vi "read_db_for_plot.vi"(8 "error in (no error)":errorcluster, 11 "Constraints 2":T1={"Upper Timestamp Range"=timestamp(0 s since 1904-01-01), "Lower Timestamp Range"=timestamp(0 s since 1904-01-01), "Experiment Group:"="", "Experiment Name:"=[], "Upper Velocity Limit (km/s)"=0.0, "Lower Velocity Limit (km/s)"=0.0, "Upper Mass Limit (kg)"=0.0, "Lower Mass Limit (kg)"=0.0, "Estimate Source "=-2, "name array"=[]} {"Estimate Source" items=["Any Source."=-2, "No Shot"=-1, "Basic Labview Estimate"=0, "IDL Estimate From Andrew"=1, "IDL Estimate From Tobin"=2, "Old Metadata"=3]}) -> (0 "error out":errorcluster, 1 "Total Number of events":i64, 2 "Dust Event ID Array":i64[](array[numeric]), 3 "Dust Array":T3[](array[typedef]) {"File Location" items=["Currently Writing"=-3, "Labview Files"=-2, "Mars Data Processing Factility"=-1, "Local Cache "=0, "Old Storage"=1, "Storage"=2]; "Estimate Source" items=["Any Source."=-2, "No Shot"=-1, "Basic Labview Estimate"=0, "IDL Estimate From Andrew"=1, "IDL Estimate From Tobin"=2, "Old Metadata"=3]}, 4 "Dust Info":cluster{"Density":dbl, "Name":string}[](array[cluster]))   [LabVIEW 2012]
uses:
  Public API/Query_Dust_Event.ctl
  Estimate_source.ctl
  File_location.ctl
  Constraints.ctl
  <vilib>/addons/database/Auxilliary.llb/DB Tools Cursor Type.ctl
  <vilib>/addons/database/Connection.llb/Conn Execute.vi
  <vilib>/addons/database/Recordset.llb/Rec Fetch Recordset Data (R).vi
  <vilib>/addons/database/Recordset.llb/Rec Destroy - Connection.vi
  <vilib>/addons/database/_DB Variant To Data/Database Variant To Data.xnode
  <vilib>/addons/database/NI_Database_API.lvlib
panel:
  out "resulting string":string
  out "SQL Query Sintax":string
  # "Dust Event"
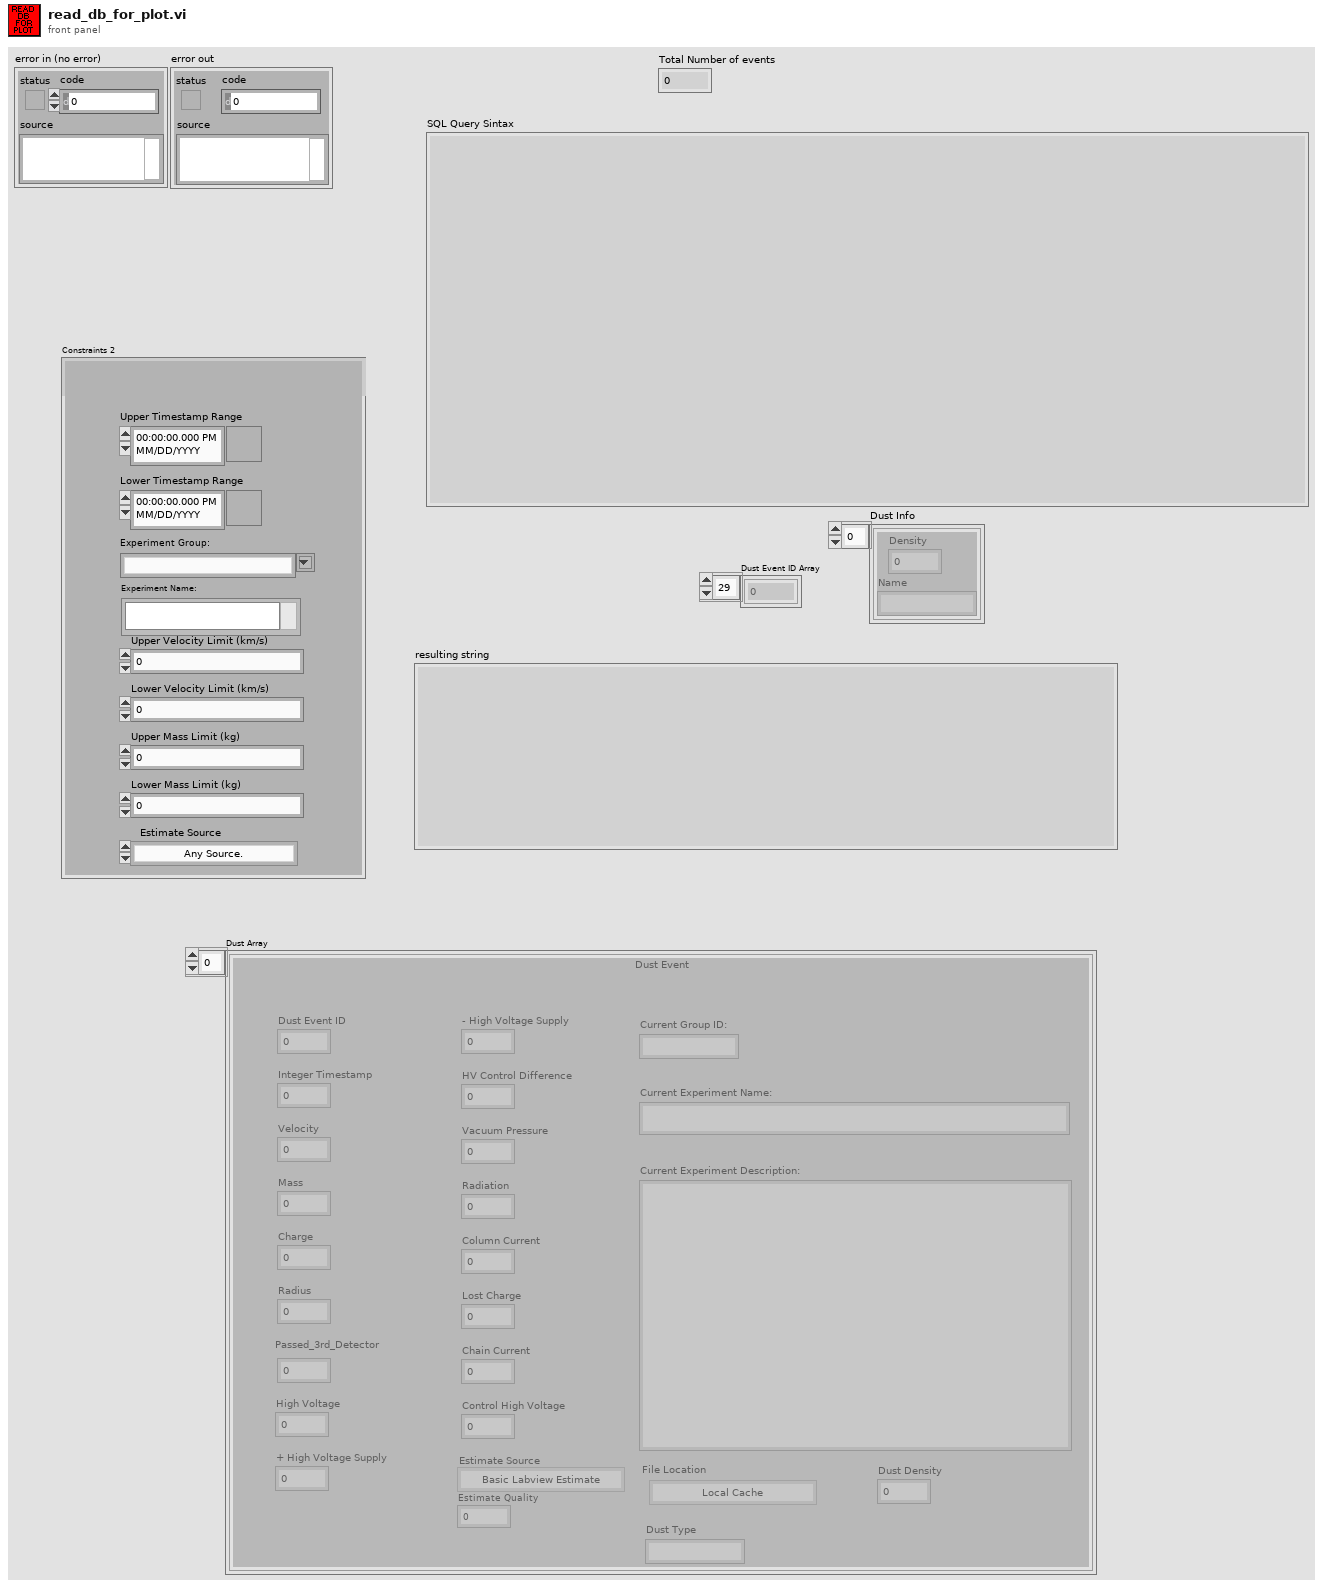
[diagram p1: front panel]
types:
  T1 = typedef "Constraints.ctl" = cluster{"Upper Timestamp Range":timestamp, "Lower Timestamp Range":timestamp, "Experiment Group:":string, "Experiment Name:":i32[], "Upper Velocity Limit (km/s)":dbl, "Lower Velocity Limit (km/s)":dbl, "Upper Mass Limit (kg)":dbl, "Lower Mass Limit (kg)":dbl, "Estimate Source ":T2, "name array":string[]}
  T2 = typedef "Estimate_source.ctl" = i8
  T3 = typedef "Query_Dust_Event.ctl" = cluster{"Dust Event ID":i64, "Integer Timestamp":i64, "Velocity":sgl, "Mass":sgl, "Charge":sgl, "Radius":sgl, "Passed_3rd_Detector":i8, "High Voltage":sgl, "+ High Voltage Supply":sgl, "- High Voltage Supply":sgl, "HV Control Difference":sgl, "Vacuum Pressure":sgl, "Radiation":sgl, "Column Current":sgl, "Lost Charge":sgl, "Chain Current":sgl, "Control High Voltage":sgl, "Current Group ID:":string, "Current Experiment Name:":string, "Current Experiment Description:":string, "Estimate Source":T2, "Estimate Quality":sgl, "File Location":T4, "Dust Type":string, "Dust Density":sgl}
  T4 = typedef "File_location.ctl" = i8
  T5 = typedef "NI_Database_API.lvlib/DB Tools Cursor Type.ctl" = enum16{"forward-only", "keyset", "dynamic", "static"}
  T6 = typedef "NI_Database_API.lvlib/Conn ObjectReference.ctl" = refnum<k1>
  T7 = typedef "NI_Database_API.lvlib/Rec ObjectReference.ctl" = refnum<k1>
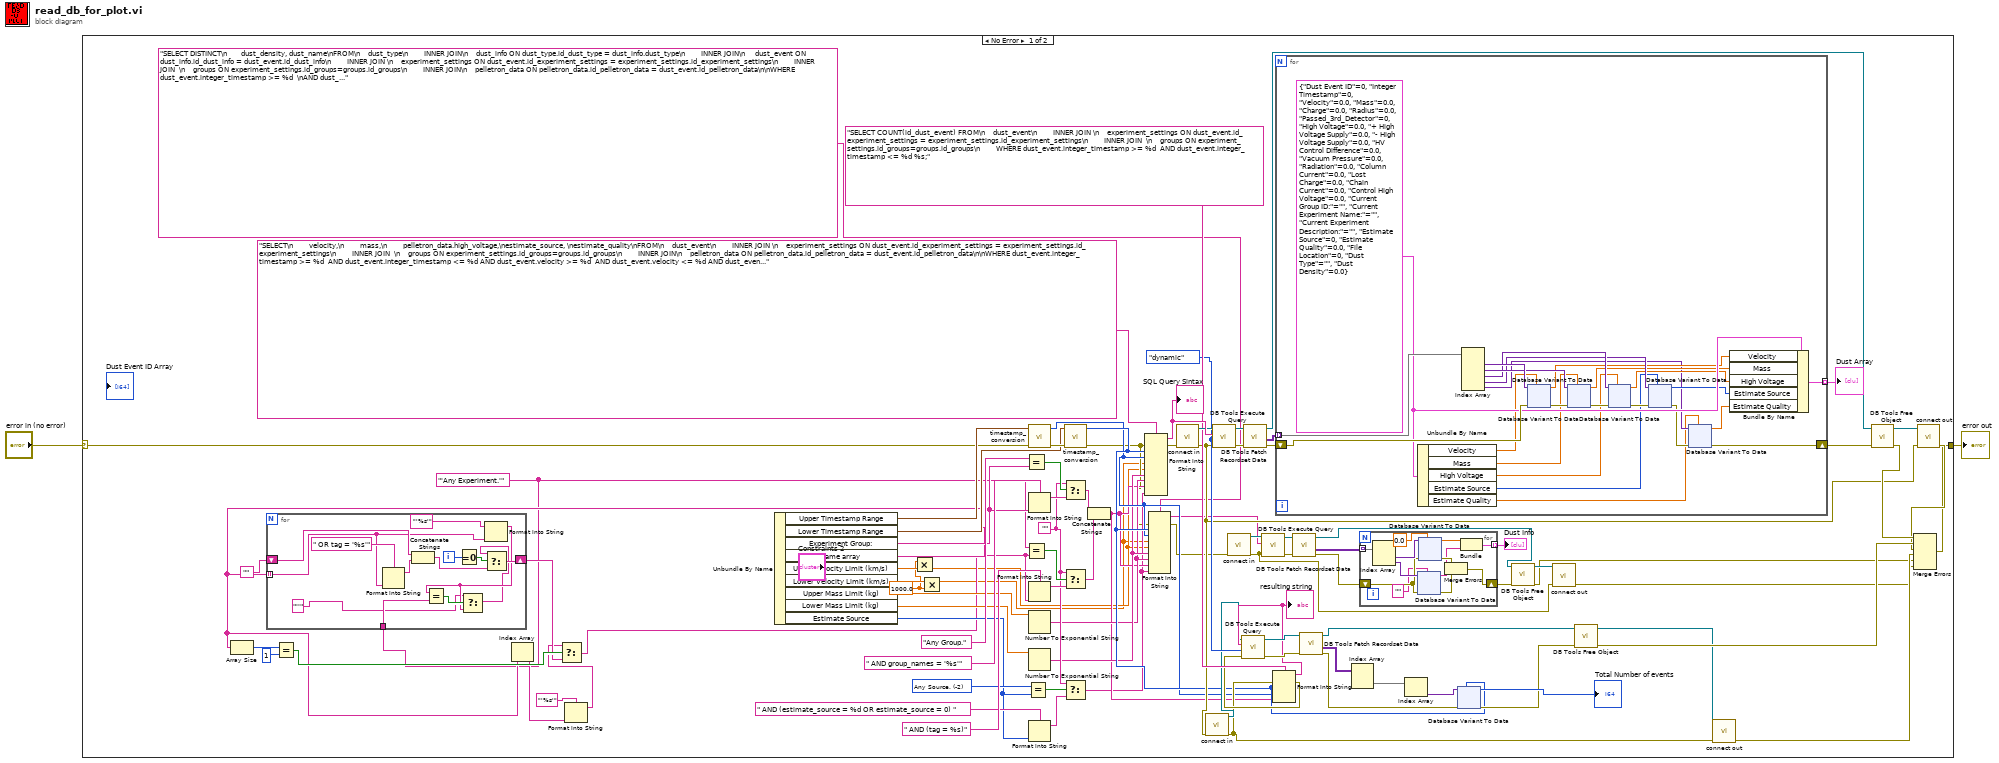
[diagram p0: block diagram]
diagram:
  n1 = case shown="No Error" "error in (no error)" {
    selector: "error in (no error)" -> [w65 w404]
    tunnel: [w47 w404] -> w1
    frame No Error {
      w3 = 1000.0 ("y")
      w74 = T2 -2 items=["Any Source."=-2, "No Shot"=-1, "Basic Labview Estimate"=0, "IDL Estimate From Andrew"=1, "IDL Estimate From Keith"=2, "Old Metadata"=3] ("Estimate Source")
      w70 = ""
      w53 = "'Any Experiment.'"
      w41 = DB_Tools_Cursor_Type."dynamic" ("cursor type")
      n2 = Unbundle By Name("Constraints 2") -> ("Upper Timestamp Range"=w84:timestamp, "Lower Timestamp Range"=w85:timestamp, "Experiment Group:"=w81:string, "name array"=w58:string[], "Upper Velocity Limit (km/s)"=w26:dbl, "Lower Velocity Limit (km/s)"=w27:dbl, "Upper Mass Limit (kg)"=w77:dbl, "Lower Mass Limit (kg)"=w76:dbl, "Estimate Source"=w73:T2)
      n3 = Array Size(array=w58) -> (size(s)=w63:i32)
      n4 = for {
        tunnel: w58 -> [w212] mode=indexing
        shift-right: [w214] -> w59
        shift-left: "" -> [w219]
        tunnel: w53 -> [w210]
        i -> [w216]
        n5 = Format Into String(format string=" OR tag = '%s'" ("string"), w212) -> (resulting string=w218:string)  [unwired: 2 in, 1 out]
        n6 = Concatenate Strings(w219, w218) -> (w213:string)
        n7 = Equal To 0?(x=w216) -> (x = 0?=w215:bool)
        n8 = Format Into String(format string="'%s'", w212) -> (resulting string=w208:string)  [unwired: 2 in, 1 out]
        n9 = Equal?(x=w208, y=w210) -> (x = y?=w209:bool)
        n10 = Select(t="''", s=w209, f=w208) -> (s? t:f=w207:string)
        n11 = Select(t=w207, s=w215, f=w213) -> (s? t:f=w214:string)
      }
      n12 = Equal?(x=w63, y=1) -> (x = y?=w61:bool)
      n13 = Index Array(array=w58) -> (element=w56:string)  [unwired: 1 in]
      n14 = Format Into String(format string="'%s'", w56) -> (resulting string=w55:string)  [unwired: 2 in, 1 out]
      n15 = Select(t=w55, s=w61, f=w59) -> (s? t:f=w54:string)
      n16 = Multiply(x=w3, y=w26) -> (x*y=w5:dbl)
      n17 = Multiply(x=w27, y=w3) -> (x*y=w4:dbl)
      n18 = Equal?(x="Any Group.", y=w81) -> (x = y?=w90:bool)
      n19 = Equal?(x=w53, y=w54) -> (x = y?=w91:bool)
      n20 = Equal?(x=w74, y=w73) -> (x = y?=w72:bool)
      n21 = call "timestamp_conversion.vi"("error in (no error)"=w65, "Time Stamp"=w84) -> ("error out"=w89:errorcluster, "Integer Time"=w28:i64)  [unwired: 7 in]
      n22 = Format Into String(format string=" AND group_names = '%s'" ("string"), w81) -> (resulting string=w80:string)  [unwired: 2 in, 1 out]
      n23 = Format Into String(format string=" AND (tag = %s)" ("string"), w54) -> (resulting string=w78:string)  [unwired: 2 in, 1 out]
      n24 = Number To Exponential String(number=w77) -> (E-format string=w24:string)  [unwired: 3 in]
      n25 = Number To Exponential String(number=w76) -> (E-format string=w25:string)  [unwired: 3 in]
      n26 = Format Into String(format string=" AND (estimate_source = %d OR estimate_source = 0) " ("string"), w73) -> (resulting string=w71:string)  [unwired: 2 in, 1 out]
      n27 = call "timestamp_conversion.vi"("error in (no error)"=w89, "Time Stamp"=w85) -> ("error out"=w20:errorcluster, "Integer Time"=w29:i64)  [unwired: 7 in]
      n28 = Select(t=w70, s=w90, f=w80) -> (s? t:f=w86:string)
      n29 = Select(t=w70, s=w91, f=w78) -> (s? t:f=w87:string)
      n30 = Select(t=w70, s=w72, f=w71) -> (s? t:f=w22:string)
      n31 = Concatenate Strings(w87, w86) -> (w23:string)
      n32 = Format Into String(format string="SELECT\n        velocity,\n        mass,\n        pelletron_data.high_voltage,\nestimate_source, \nestimate_quality\nFROM\n    dust_event\n        INNER JOIN \n    experiment_settings ON dust_event.id_experiment_settings = experiment_settings.id_experiment_settings\n        INNER JOIN  \n    groups ON experiment_settings.id_groups=groups.id_groups\n        INNER JOIN\n    pelletron_data ON pelletron_data.id_pelletron_data = dust_event.id_pelletron_data\n\nWHERE dust_event.integer_timestamp >= %d  AND dust_event.integer_timestamp <= %d AND dust_event.velocity >= %d  AND dust_event.velocity <= %d AND dust_event.mass >= %s  AND dust_event.mass <= %s%s%s; " ("string"), error in=w20, w29, w28, w4, w5, w25, w24, w23, w22) -> (resulting string=w67:string, error out=w64:errorcluster)  [unwired: 1 in]
      "SQL Query Sintax" <- w67
      n33 = Format Into String(format string="SELECT DISTINCT\n       dust_density, dust_name\nFROM\n    dust_type\n        INNER JOIN\n    dust_info ON dust_type.id_dust_type = dust_info.dust_type\n        INNER JOIN\n     dust_event ON dust_info.id_dust_info = dust_event.id_dust_info\n        INNER JOIN \n    experiment_settings ON dust_event.id_experiment_settings = experiment_settings.id_experiment_settings\n        INNER JOIN  \n    groups ON experiment_settings.id_groups=groups.id_groups\n        INNER JOIN\n    pelletron_data ON pelletron_data.id_pelletron_data = dust_event.id_pelletron_data\n\nWHERE dust_event.integer_timestamp >= %d  \nAND dust_event.integer_timestamp <= %d AND dust_event.velocity >= %d  AND dust_event.velocity <= %d AND dust_event.mass >= %s  AND dust_event.mass <= %s%s%s; " ("string"), error in=w20, w29, w28, w4, w5, w25, w24, w23, w22) -> (resulting string=w17:string, error out=w19:errorcluster)  [unwired: 1 in]
      n34 = call "connect in.vi"("error in (no error)"=w64) -> ("error out"=w34:errorcluster, "Database Connection"=w51:T6)  [unwired: 6 in, 1 out]
      n35 = call "connect in.vi"("error in (no error)"=w34) -> ("error out"=w32:errorcluster, "Database Connection"=w33:T6)  [unwired: 6 in, 1 out]
      n36 = call-poly <vilib>:"DB Tools Execute Query.vi"("error in (no error)"=w34, "cursor type"=w41, "SQL query"=w67, "connection reference"=w51) -> ("error out"=w69:errorcluster, "recordset reference"=w68:T7)  [unwired: 4 in]
      n37 = call "connect in.vi"("error in (no error)"=w19) -> ("error out"=w8:errorcluster, "Database Connection"=w18:T6)  [unwired: 6 in, 1 out]
      n38 = call-poly <vilib>:"DB Tools Fetch Recordset Data.vi"("error in (no error)"=w69, "recordset reference"=w68) -> ("error out"=w96:errorcluster, "recordset data"=w93:variant[][], "recordset reference out"=w97:T7)  [unwired: 3 in]
      n39 = call-poly <vilib>:"DB Tools Execute Query.vi"("error in (no error)"=w8, "SQL query"=w17, "connection reference"=w18) -> ("error out"=w15:errorcluster, "recordset reference"=w16:T7)  [unwired: 5 in]
      n40 = Format Into String(format string="SELECT COUNT(id_dust_event) FROM\n    dust_event\n        INNER JOIN \n    experiment_settings ON dust_event.id_experiment_settings = experiment_settings.id_experiment_settings\n        INNER JOIN  \n    groups ON experiment_settings.id_groups=groups.id_groups\n        WHERE dust_event.integer_timestamp >= %d  AND dust_event.integer_timestamp <= %d %s;" ("SQL query"), error in=w32, w29, w28, w23) -> (resulting string=w43:string, error out=w42:errorcluster)  [unwired: 1 in]
      "resulting string" <- w43
      n41 = call-poly <vilib>:"DB Tools Execute Query.vi"("error in (no error)"=w42, "cursor type"=w41, "SQL query"=w43, "connection reference"=w33) -> ("error out"=w52:errorcluster, "recordset reference"=w46:T7)  [unwired: 4 in]
      n42 = for {
        tunnel: w93 -> [w243] mode=indexing
        shift-right: [w233] -> w95
        shift-left: w96 -> [w242]
        tunnel: [w232] -> w92 mode=indexing
        w240 = T3 {"Dust Event ID"=0, "Integer Timestamp"=0, "Velocity"=0.0, "Mass"=0.0, "Charge"=0.0, "Radius"=0.0, "Passed_3rd_Detector"=0, "High Voltage"=0.0, "+ High Voltage Supply"=0.0, "- High Voltage Supply"=0.0, "HV Control Difference"=0.0, "Vacuum Pressure"=0.0, "Radiation"=0.0, "Column Current"=0.0, "Lost Charge"=0.0, "Chain Current"=0.0, "Control High Voltage"=0.0, "Current Group ID:"="", "Current Experiment Name:"="", "Current Experiment Description:"="", "Estimate Source"=0, "Estimate Quality"=0.0, "File Location"=0, "Dust Type"="", "Dust Density"=0.0} ("Cluster")
        n43 = Unbundle By Name(w240) -> ("Velocity"=w231:sgl, "Mass"=w229:sgl, "High Voltage"=w227:sgl, "Estimate Source"=w225:T2, "Estimate Quality"=w221:sgl)
        n44 = Index Array(array=w243) -> (element #1=w241:variant, element #2=w239:variant, element #3=w237:variant, element #4=w235:variant, element #5=w223:variant)  [unwired: 5 in]
        n45 = xnode "Database Variant To Data"("database variant"=w241, "error in"=w242, "type"=w231) -> ("data"=w230:sgl, "error out"=w238:errorcluster)
        n46 = xnode "Database Variant To Data"("database variant"=w239, "error in"=w238, "type"=w229) -> ("data"=w228:sgl, "error out"=w236:errorcluster)
        n47 = xnode "Database Variant To Data"("database variant"=w237, "error in"=w236, "type"=w227) -> ("data"=w226:sgl, "error out"=w234:errorcluster)
        n48 = xnode "Database Variant To Data"("database variant"=w235, "error in (no error)"=w234, "type"=w225) -> ("data"=w224:T2, "error out"=w222:errorcluster)
        n49 = xnode "Database Variant To Data"("database variant"=w223, "error in"=w222, "type"=w221) -> ("data"=w220:sgl, "error out"=w233:errorcluster)
        n50 = Bundle By Name(cluster=w240, "Velocity"=w230, "Mass"=w228, "High Voltage"=w226, "Estimate Source"=w224, "Estimate Quality"=w220) -> (w232:T3)
      }
      "Dust Array" <- w92
      n51 = call-poly <vilib>:"DB Tools Fetch Recordset Data.vi"("error in (no error)"=w15, "recordset reference"=w16) -> ("error out"=w13:errorcluster, "recordset data"=w14:variant[][], "recordset reference out"=w10:T7)  [unwired: 3 in]
      n52 = call-poly <vilib>:"DB Tools Fetch Recordset Data.vi"("error in (no error)"=w52, "recordset reference"=w46) -> ("error out"=w36:errorcluster, "recordset data"=w40:variant[][], "recordset reference out"=w45:T7)  [unwired: 3 in]
      n53 = Index Array(array=w40) -> (element=w39:variant[])  [unwired: 2 in]
      n54 = for {
        tunnel: w14 -> [w109] mode=indexing
        shift-right: [w103] -> w11
        shift-left: w13 -> [w106]
        tunnel: [w98] -> w12 mode=indexing
        n55 = Index Array(array=w109) -> (element #1=w108:variant, element #2=w107:variant)  [unwired: 2 in]
        n56 = xnode "Database Variant To Data"("database variant"=w107, "error in (no error)"=w106, "type"="") -> ("data"=w99:string, "error out"=w105:errorcluster)
        n57 = xnode "Database Variant To Data"("database variant"=w108, "error in (no error)"=w106, "type"=0.0) -> ("data"=w100:dbl, "error out"=w104:errorcluster)
        n58 = Merge Errors(w104, w105) -> (w103:errorcluster)
        n59 = Bundle("data"=w100, "data"=w99) -> (w98:cluster{"data":dbl, "data":string})  [unwired: 1 in]
      }
      "Dust Info" <- w12
      n60 = Index Array(array=w39) -> (element=w38:variant)  [unwired: 1 in]
      n61 = xnode "Database Variant To Data"("database variant"=w38, "error in (no error)"=w36, "type"=w29) -> ("data"=→"Total Number of events":i64, "error out"=w35:errorcluster)
      n62 = call-poly <vilib>:"DB Tools Free Object.vi"("error in (no error)"=w11, "recordset reference"=w10) -> ("error out"=w7:errorcluster, "connection reference"=w9:T6)  [unwired: 8 in]
      n63 = call "connect out.vi"("error in (no error)"=w8, "connection reference"=w9) -> ("error out"=w6:errorcluster)  [unwired: 9 in]
      n64 = call-poly <vilib>:"DB Tools Free Object.vi"("error in (no error)"=w35, "recordset reference"=w45) -> ("error out"=w50:errorcluster, "connection reference"=w31:T6)  [unwired: 8 in]
      n65 = call "connect out.vi"("error in (no error)"=w32, "connection reference"=w31) -> ("error out"=w30:errorcluster)  [unwired: 9 in]
      n66 = call-poly <vilib>:"DB Tools Free Object.vi"("error in (no error)"=w95, "recordset reference"=w97) -> ("error out"=w49:errorcluster, "connection reference"=w94:T6)  [unwired: 8 in]
      n67 = call "connect out.vi"("error in (no error)"=w34, "connection reference"=w94) -> ("error out"=w48:errorcluster)  [unwired: 9 in]
      n68 = Merge Errors(w49, w50, w48, w30, w7, w6) -> (w47:errorcluster)
    }
    frame Error {
    }
  }
  "error out" <- w1
